vi "StaticCalibration2.vi"(0 "SENSOR":T1, 11 "error in (no error)":errorcluster caption="错误输入（无错误）") -> (4 "Vres":dbl, 6 "Angle out":dbl, 8 "Vres_FD":i32, 10 "OK？":bool, 15 "error out":errorcluster caption="错误输出")   [LabVIEW 2020]
doc: "该模板用于创建子VI。"
uses:
  Global_Variable/Global.vi
  <userlib>/DAQNavi Polymorphic VI/create/DAQNavi Create Channel.vi
  <userlib>/DAQNavi Polymorphic VI/create/DAQNavi Create Channel(CI-PulseWidth).vi
  <userlib>/DAQNavi Polymorphic VI/read/DAQNavi Read.vi
  <userlib>/DAQNavi Polymorphic VI/read/DAQNavi Read (Counter Pulse Width 1Chan 1Samp).vi
  <userlib>/DAQNavi Polymorphic VI/configure/task/DAQNavi Clear Task.vi
  <userlib>/_MGI/1D Array/MGI Average.vi
  <userlib>/_MGI/1D Array/MGI Average/MGI Average (DBL[]).vi
panel:
  out "T2(%)":dbl
  out "T1(%)":dbl
  out "S(%)":dbl
  out "P(%)":dbl
  out "T2ROC_1+T2ROC_2":i32
  out "T1ROC_1+T1ROC_2":i32
  out "PROC_1":i32
  out "T2ROC_1":i32
  out "T1ROC_1":i32
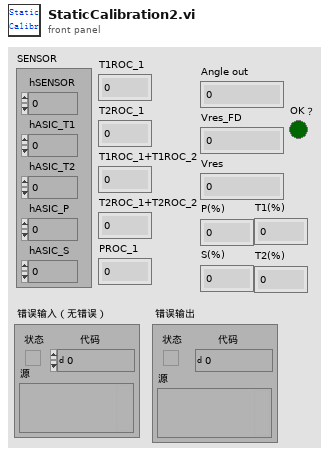
[diagram p1: front panel]
types:
  T1 = cluster{"hSENSOR":i32, "hASIC_T1":i32, "hASIC_T2":i32, "hASIC_P":i32, "hASIC_S":i32}
  T2 = cluster{"主信号":cluster{"单位":string, "下限":dbl, "上限":dbl}, "副信号":cluster{"单位":string, "下限":dbl, "上限":dbl}, "主副和":cluster{"单位":string, "下限":dbl, "上限":dbl}, "主副差":cluster{"单位":string, "下限":dbl, "上限":dbl}, "Vres":cluster{"单位":string, "下限":dbl, "上限":dbl}}
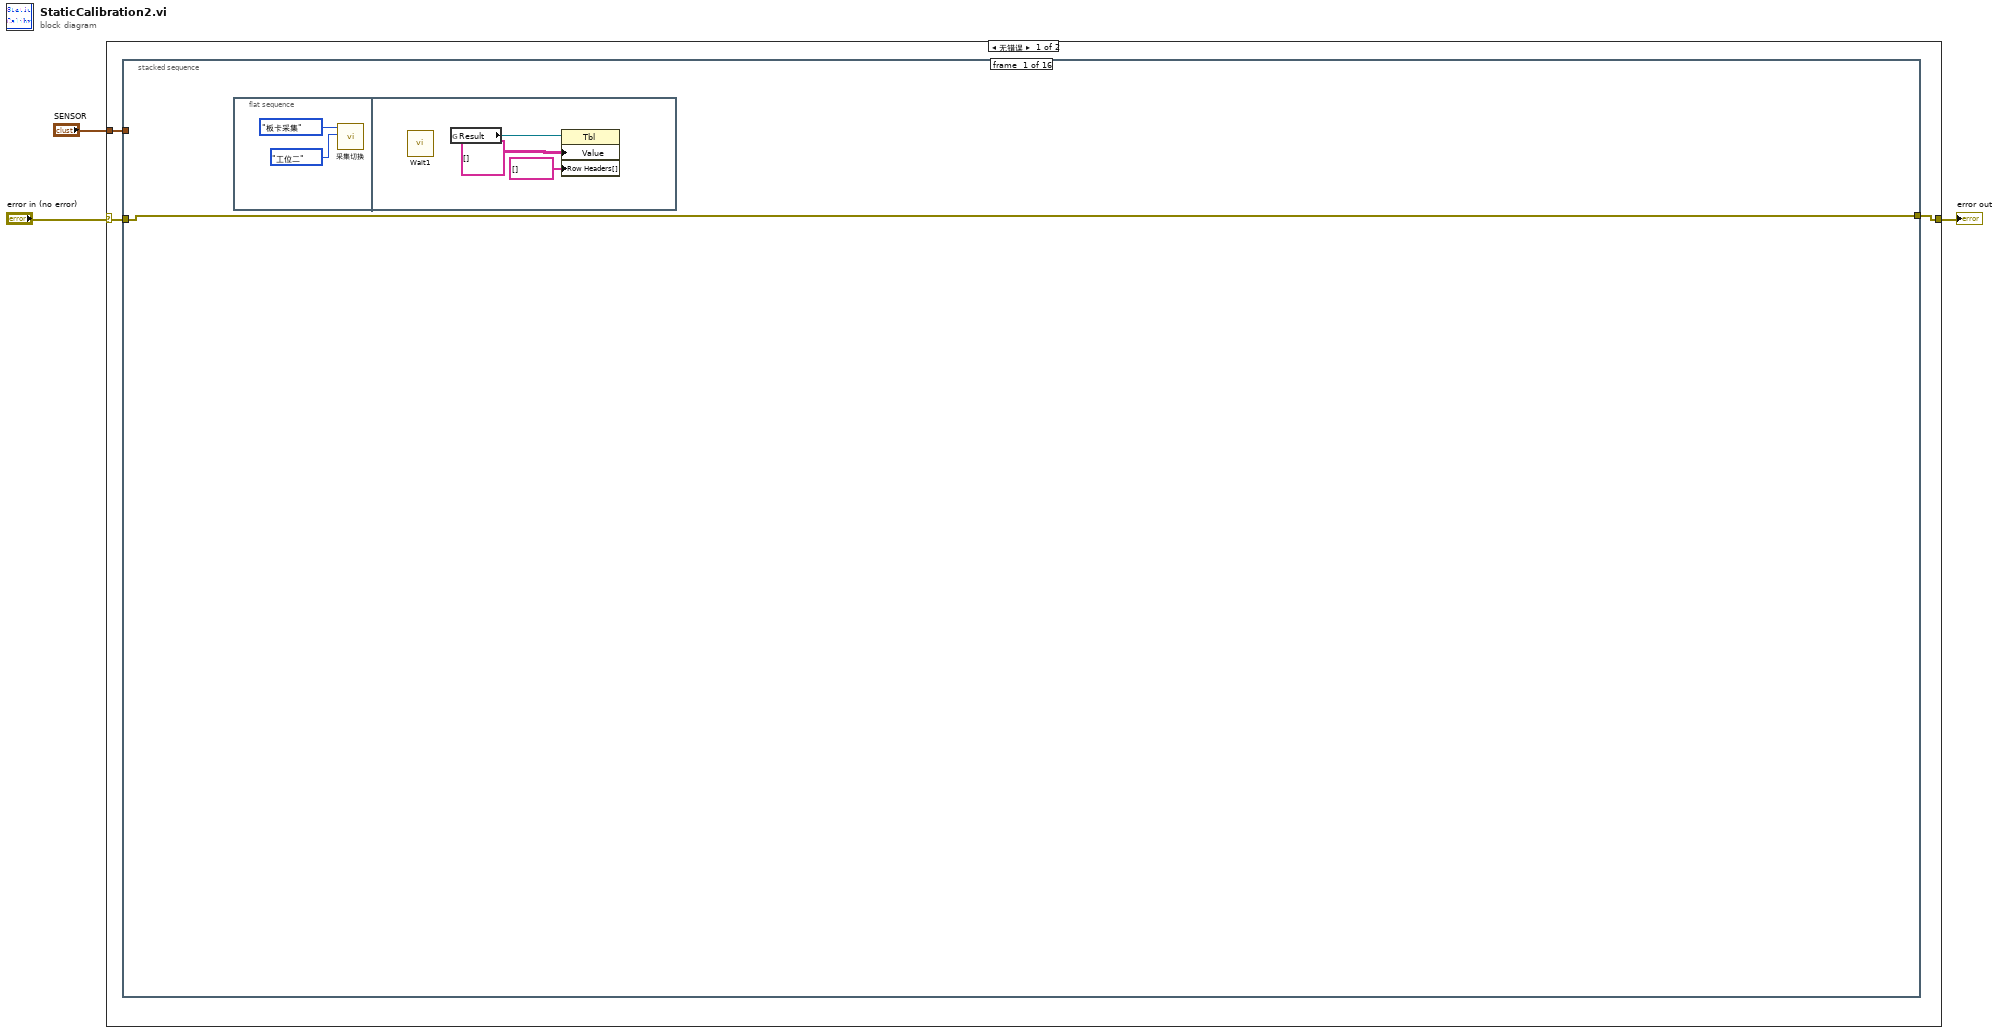
[diagram p0: block diagram]
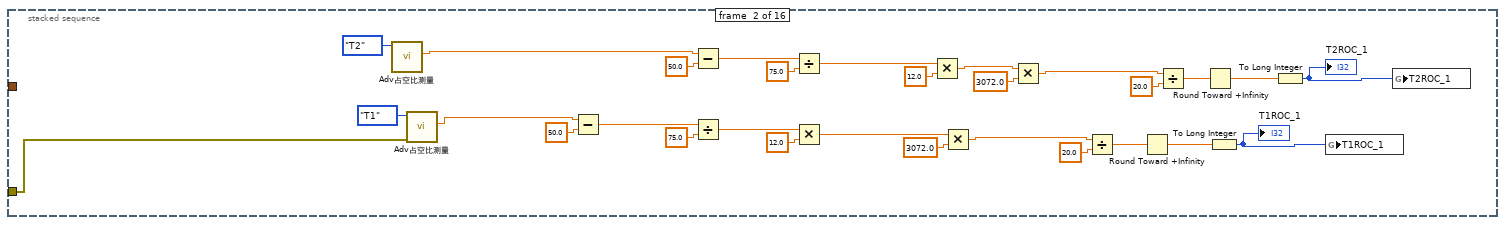
[diagram p2: hidden frame]
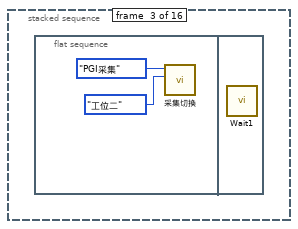
[diagram p3: hidden frame]
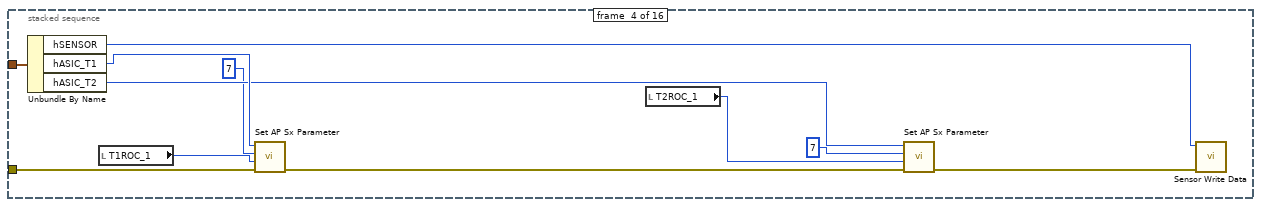
[diagram p4: hidden frame]
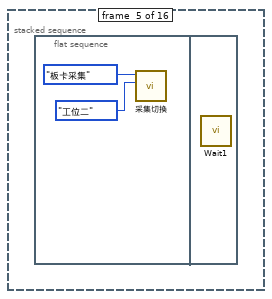
[diagram p5: hidden frame]
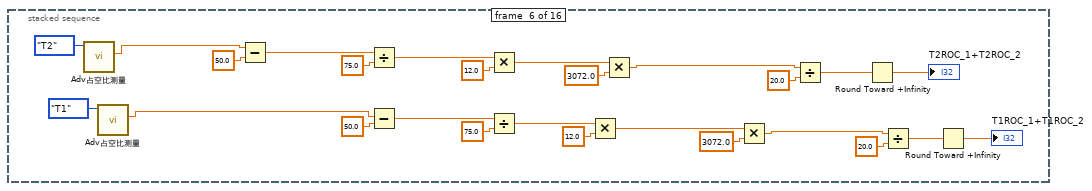
[diagram p6: hidden frame]
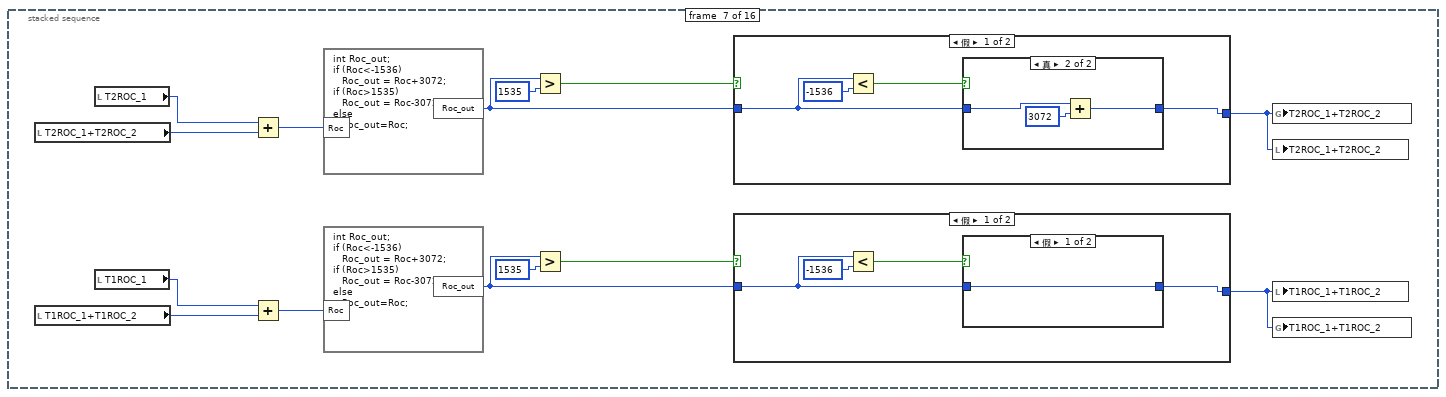
[diagram p7: hidden frame]
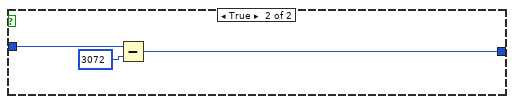
[diagram p9: hidden frame]
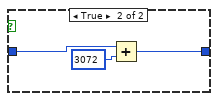
[diagram p10: hidden frame]
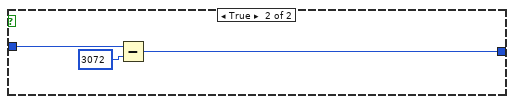
[diagram p11: hidden frame]
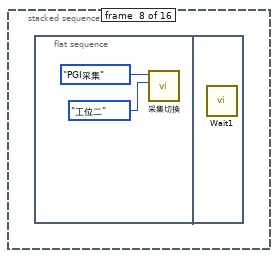
[diagram p12: hidden frame]
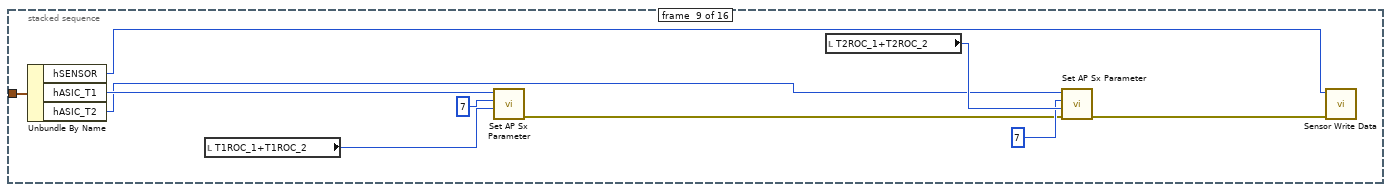
[diagram p13: hidden frame]
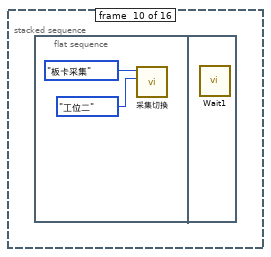
[diagram p14: hidden frame]
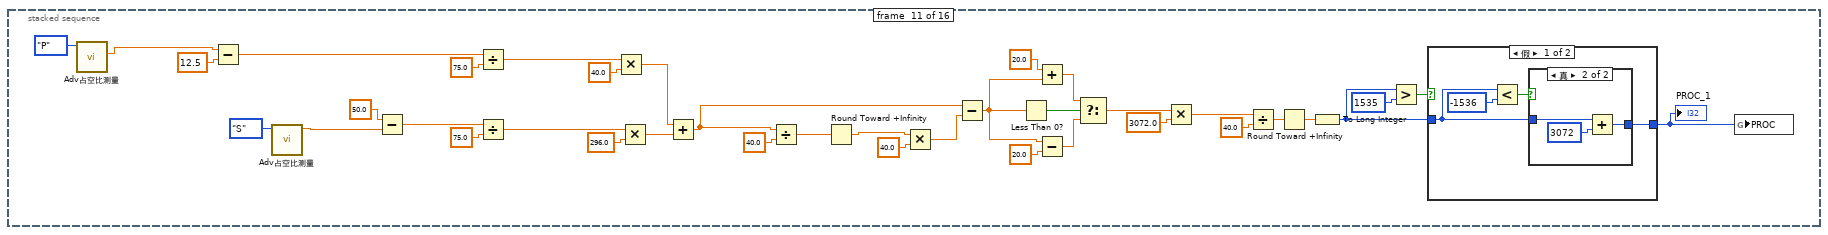
[diagram p15: hidden frame]
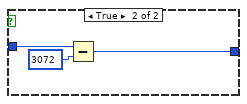
[diagram p17: hidden frame]
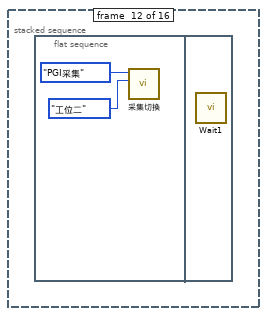
[diagram p18: hidden frame]
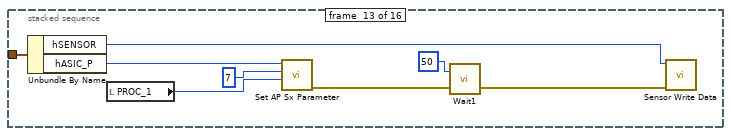
[diagram p19: hidden frame]
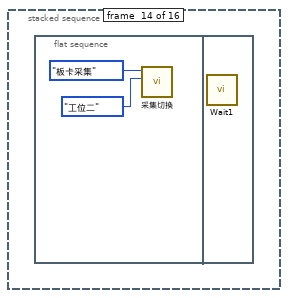
[diagram p20: hidden frame]
diagram:
  n1 = case shown="无错误" "error in (no error)" {
    selector: "error in (no error)" -> [w5 w304]
    tunnel: [w4 w304] -> w2
    tunnel: "SENSOR" -> [w6 _]
    frame No Error {
      n2 = stacked-sequence {
        tunnel: w6 -> [_ _ _ w52 _ _ _ _ w129 _ _ _ w186 _ _ _]
        tunnel: w5 -> [w7 w13 _ w44 _ _ _ _ _ _ _ _ _ _ _ _]
        tunnel: [w7 _ _ _ _ _ _ _ _ _ _ _ _ _ _ _] -> w4
        frame #0 {
          n3 = flat-sequence {
            frame #0 {
              n4 = call "采集切换.vi"("工位"=enum16{"工位一", "工位二"}."工位二", "采集方式"=enum16{"板卡采集", "PGI采集"}."板卡采集") -> ()  [unwired: 10 in]
            }
            frame #1 {
              n5 = call "Wait1.vi"() -> ()  [unwired: 3 in, 1 out]
              n6 = global read "Global.vi" "Result"() -> (w12:refnum<vi>)
              n7 = property class="Tbl"(reference=w12, "Value"=string[][] [] ("值"), "Row Headers[]"=string[] [] ("行首字符串[]")) -> ()  [unwired: 1 in, 2 out]
            }
          }
        }
        frame #1 {
          n8 = call "Adv占空比测量.vi"("通道"=enum16{"T1", "T2", "P", "S"}."T2") -> ("占空比2"=w16:dbl)  [unwired: 5 in, 4 out]
          n9 = call "Adv占空比测量.vi"("通道"=enum16{"T1", "T2", "P", "S"}."T1", "error in (no error)"=w13) -> ("占空比2"=w14:dbl)  [unwired: 4 in, 4 out]
          n10 = Subtract(x=w14, y=50.0) -> (x-y=w40:dbl)
          n11 = Subtract(x=w16, y=50.0) -> (x-y=w25:dbl)
          n12 = Divide(x=w40, y=75.0) -> (x/y=w38:dbl)
          n13 = Divide(x=w25, y=75.0) -> (x/y=w27:dbl)
          n14 = Multiply(x=w38, y=12.0) -> (x*y=w36:dbl)
          n15 = Multiply(x=w27, y=12.0) -> (x*y=w29:dbl)
          n16 = Multiply(x=w36, y=3072.0) -> (x*y=w34:dbl)
          n17 = Multiply(x=w29, y=3072.0) -> (x*y=w31:dbl)
          n18 = Divide(x=w34, y=20.0) -> (x/y=w23:dbl)
          n19 = Round Toward +Infinity(x=w23) -> (ceil(x): smallest int >= x=w21:dbl)
          n20 = Divide(x=w31, y=20.0) -> (x/y=w22:dbl)
          n21 = Round Toward +Infinity(x=w22) -> (ceil(x): smallest int >= x=w20:dbl)
          n22 = To Long Integer(number=w21) -> (32bit integer=w18:i32)
          "T1ROC_1" <- w18
          n23 = To Long Integer(number=w20) -> (32bit integer=w19:i32)
          "T2ROC_1" <- w19
          n24 = global write "Global.vi" "T1ROC_1"(w18) -> ()
          n25 = global write "Global.vi" "T2ROC_1"(w19) -> ()
        }
        frame #2 {
          n26 = flat-sequence {
            frame #0 {
              n27 = call "采集切换.vi"("工位"=enum16{"工位一", "工位二"}."工位二", "采集方式"=enum16{"板卡采集", "PGI采集"}."PGI采集") -> ()  [unwired: 10 in]
            }
            frame #1 {
              n28 = call "Wait1.vi"() -> ()  [unwired: 3 in, 1 out]
            }
          }
        }
        frame #3 {
          n29 = Unbundle By Name(w52) -> ("hSENSOR"=w49:i32, "hASIC_T1"=w51:i32, "hASIC_T2"=w50:i32)
          n30 = local read "T1ROC_1"() -> (w53:i32)
          n31 = call "Set AP Sx Parameter.vi"("error in (no error)"=w44, "para2"=w53, "asicBitsName"=7, "asicHandle"=w51) -> ("error out"=w46:errorcluster)  [unwired: 6 in, 1 out]
          n32 = local read "T2ROC_1"() -> (w54:i32)
          n33 = call "Set AP Sx Parameter.vi"("error in (no error)"=w46, "para2"=w54, "asicBitsName"=7, "asicHandle"=w50) -> ("error out"=w45:errorcluster)  [unwired: 6 in, 1 out]
          n34 = call "Sensor Write Data.vi"("error in (no error)"=w45, "sensorHandle"=w49) -> ()  [unwired: 8 in, 2 out]
        }
        frame #4 {
          n35 = flat-sequence {
            frame #0 {
              n36 = call "采集切换.vi"("工位"=enum16{"工位一", "工位二"}."工位二", "采集方式"=enum16{"板卡采集", "PGI采集"}."板卡采集") -> ()  [unwired: 10 in]
            }
            frame #1 {
              n37 = call "Wait1.vi"() -> ()  [unwired: 3 in, 1 out]
            }
          }
        }
        frame #5 {
          n38 = call "Adv占空比测量.vi"("通道"=enum16{"T1", "T2", "P", "S"}."T2") -> ("占空比2"=w60:dbl)  [unwired: 5 in, 4 out]
          n39 = call "Adv占空比测量.vi"("通道"=enum16{"T1", "T2", "P", "S"}."T1") -> ("占空比2"=w59:dbl)  [unwired: 5 in, 4 out]
          n40 = Subtract(x=w60, y=50.0) -> (x-y=w82:dbl)
          n41 = Divide(x=w82, y=75.0) -> (x/y=w81:dbl)
          n42 = Subtract(x=w59, y=50.0) -> (x-y=w75:dbl)
          n43 = Multiply(x=w81, y=12.0) -> (x*y=w80:dbl)
          n44 = Divide(x=w75, y=75.0) -> (x/y=w76:dbl)
          n45 = Multiply(x=w76, y=12.0) -> (x*y=w77:dbl)
          n46 = Multiply(x=w80, y=3072.0) -> (x*y=w79:dbl)
          n47 = Multiply(x=w77, y=3072.0) -> (x*y=w78:dbl)
          n48 = Divide(x=w79, y=20.0) -> (x/y=w73:dbl)
          n49 = Round Toward +Infinity(x=w73) -> (ceil(x): smallest int >= x=→"T2ROC_1+T2ROC_2":dbl)
          n50 = Divide(x=w78, y=20.0) -> (x/y=w74:dbl)
          n51 = Round Toward +Infinity(x=w74) -> (ceil(x): smallest int >= x=→"T1ROC_1+T1ROC_2":dbl)
        }
        frame #6 {
          n52 = local read "T2ROC_1+T2ROC_2"() -> (w85:i32)
          n53 = local read "T1ROC_1+T1ROC_2"() -> (w86:i32)
          n54 = local read "T2ROC_1"() -> (w93:i32)
          n55 = local read "T1ROC_1"() -> (w94:i32)
          n56 = Add(x=w93, y=w85) -> (x+y=w95:i32)
          n57 = Add(x=w94, y=w86) -> (x+y=w96:i32)
          n58 = formula code="int Roc_out;\nif (Roc<-1536)\n   Roc_out = Roc+3072;\nif (Roc>1535)\n   Roc_out = Roc-3072;\nelse\n   Roc_out=Roc;"("Roc"=w95) -> ("Roc_out"=w87:i32)
          n59 = formula code="int Roc_out;\nif (Roc<-1536)\n   Roc_out = Roc+3072;\nif (Roc>1535)\n   Roc_out = Roc-3072;\nelse\n   Roc_out=Roc;"("Roc"=w96) -> ("Roc_out"=w90:i32)
          n60 = Greater?(x=w87, y=1535) -> (0:w88:bool)
          n61 = Greater?(x=w90, y=1535) -> (0:w91:bool)
          n62 = case shown="假" w88 {
            tunnel: w87 -> [w98 w106]
            tunnel: [w97 w105] -> w83
            frame False {
              n63 = Less?(x=w98, y=-1536) -> (x < y?=w99:bool)
              n64 = case shown="真" w99 {
                tunnel: w98 -> [w101 w104]
                tunnel: [w101 w102] -> w97
                frame False {
                }
                frame True {
                  n65 = Add(x=w104, y=3072) -> (x+y=w102:i32)
                }
              }
            }
            frame True {
              n66 = Subtract(x=w106, y=3072) -> (x-y=w105:i32)
            }
          }
          n67 = case shown="假" w91 {
            tunnel: w90 -> [w109 w117]
            tunnel: [w108 w116] -> w84
            frame False {
              n68 = Less?(x=w109, y=-1536) -> (x < y?=w110:bool)
              n69 = case shown="假" w110 {
                tunnel: w109 -> [w112 w115]
                tunnel: [w112 w113] -> w108
                frame False {
                }
                frame True {
                  n70 = Add(x=w115, y=3072) -> (x+y=w113:i32)
                }
              }
            }
            frame True {
              n71 = Subtract(x=w117, y=3072) -> (x-y=w116:i32)
            }
          }
          n72 = global write "Global.vi" "T2ROC_1+T2ROC_2"(w83) -> ()
          n73 = local write "T2ROC_1+T2ROC_2"(w83) -> ()
          n74 = local write "T1ROC_1+T1ROC_2"(w84) -> ()
          n75 = global write "Global.vi" "T1ROC_1+T1ROC_2"(w84) -> ()
        }
        frame #7 {
          n76 = flat-sequence {
            frame #0 {
              n77 = call "采集切换.vi"("工位"=enum16{"工位一", "工位二"}."工位二", "采集方式"=enum16{"板卡采集", "PGI采集"}."PGI采集") -> ()  [unwired: 10 in]
            }
            frame #1 {
              n78 = call "Wait1.vi"() -> ()  [unwired: 3 in, 1 out]
            }
          }
        }
        frame #8 {
          n79 = Unbundle By Name(w129) -> ("hSENSOR"=w126:i32, "hASIC_T1"=w128:i32, "hASIC_T2"=w127:i32)
          n80 = local read "T1ROC_1+T1ROC_2"() -> (w125:i32)
          n81 = call "Set AP Sx Parameter.vi"("para2"=w125, "asicBitsName"=7, "asicHandle"=w128) -> ("error out"=w122:errorcluster)  [unwired: 7 in, 1 out]
          n82 = local read "T2ROC_1+T2ROC_2"() -> (w130:i32)
          n83 = call "Set AP Sx Parameter.vi"("error in (no error)"=w122, "para2"=w130, "asicBitsName"=7, "asicHandle"=w127) -> ("error out"=w121:errorcluster)  [unwired: 6 in, 1 out]
          n84 = call "Sensor Write Data.vi"("error in (no error)"=w121, "sensorHandle"=w126) -> ()  [unwired: 8 in, 2 out]
        }
        frame #9 {
          n85 = flat-sequence {
            frame #0 {
              n86 = call "采集切换.vi"("工位"=enum16{"工位一", "工位二"}."工位二", "采集方式"=enum16{"板卡采集", "PGI采集"}."板卡采集") -> ()  [unwired: 10 in]
            }
            frame #1 {
              n87 = call "Wait1.vi"() -> ()  [unwired: 3 in, 1 out]
            }
          }
        }
        frame #10 {
          n88 = call "Adv占空比测量.vi"("通道"=enum16{"T1", "T2", "P", "S"}."P") -> ("占空比2"=w136:dbl)  [unwired: 5 in, 4 out]
          n89 = Subtract(x=w136, y=12.5) -> (x-y=w169:dbl)
          n90 = call "Adv占空比测量.vi"("通道"=enum16{"T1", "T2", "P", "S"}."S") -> ("占空比1"=w134:dbl)  [unwired: 5 in, 4 out]
          n91 = Subtract(x=50.0, y=w134) -> (x-y=w163:dbl)
          n92 = Divide(x=w169, y=75.0) -> (x/y=w167:dbl)
          n93 = Divide(x=w163, y=75.0) -> (x/y=w161:dbl)
          n94 = Multiply(x=w167, y=40.0) -> (x*y=w165:dbl)
          n95 = Multiply(x=w161, y=296.0) -> (x*y=w159:dbl)
          n96 = Add(x=w165, y=w159) -> (x+y=w153:dbl)
          n97 = Divide(x=w153, y=40.0) -> (x/y=w157:dbl)
          n98 = Round Toward +Infinity(x=w157) -> (ceil(x): smallest int >= x=w155:dbl)
          n99 = Multiply(x=w155, y=40.0) -> (x*y=w154:dbl)
          n100 = Subtract(x=w153, y=w154) -> (x-y=w149:dbl)
          n101 = Less Than 0?(x=w149) -> (x < 0?=w148:bool)
          n102 = Add(x=20.0, y=w149) -> (x+y=w151:dbl)
          n103 = Subtract(x=w149, y=20.0 ("x")) -> (x-y=w147:dbl)
          n104 = Select(t=w151, s=w148, f=w147) -> (s? t:f=w146:dbl)
          n105 = Multiply(x=w146, y=3072.0) -> (x*y=w144:dbl)
          n106 = Divide(x=w144, y=40.0) -> (x/y=w139:dbl)
          n107 = Round Toward +Infinity(x=w139) -> (ceil(x): smallest int >= x=w138:dbl)
          n108 = To Long Integer(number=w138) -> (32bit integer=w142:i32)
          n109 = Greater?(x=w142, y=1535) -> (0:w140:bool)
          n110 = case shown="假" w140 {
            tunnel: w142 -> [w172 w180]
            tunnel: [w171 w179] -> w137
            frame False {
              n111 = Less?(x=w172, y=-1536) -> (x < y?=w173:bool)
              n112 = case shown="真" w173 {
                tunnel: w172 -> [w175 w178]
                tunnel: [w175 w176] -> w171
                frame False {
                }
                frame True {
                  n113 = Add(x=w178, y=3072) -> (x+y=w176:i32)
                }
              }
            }
            frame True {
              n114 = Subtract(x=w180, y=3072) -> (x-y=w179:i32)
            }
          }
          "PROC_1" <- w137
          n115 = global write "Global.vi" "PROC"(w137) -> ()
        }
        frame #11 {
          n116 = flat-sequence {
            frame #0 {
              n117 = call "采集切换.vi"("工位"=enum16{"工位一", "工位二"}."工位二", "采集方式"=enum16{"板卡采集", "PGI采集"}."PGI采集") -> ()  [unwired: 10 in]
            }
            frame #1 {
              n118 = call "Wait1.vi"() -> ()  [unwired: 3 in, 1 out]
            }
          }
        }
        frame #12 {
          n119 = Unbundle By Name(w186) -> ("hSENSOR"=w185:i32, "hASIC_P"=w184:i32)
          n120 = local read "PROC_1"() -> (w189:i32)
          n121 = call "Set AP Sx Parameter.vi"("para2"=w189, "asicBitsName"=7, "asicHandle"=w184) -> ("error out"=w191:errorcluster)  [unwired: 7 in, 1 out]
          n122 = call "Wait1.vi"("error in (no error)"=w191, "Wait（150ms）"=u32 50) -> ("error out"=w190:errorcluster)  [unwired: 1 in]
          n123 = call "Sensor Write Data.vi"("error in (no error)"=w190, "sensorHandle"=w185) -> ()  [unwired: 8 in, 2 out]
        }
        frame #13 {
          n124 = flat-sequence {
            frame #0 {
              n125 = call "采集切换.vi"("工位"=enum16{"工位一", "工位二"}."工位二", "采集方式"=enum16{"板卡采集", "PGI采集"}."板卡采集") -> ()  [unwired: 10 in]
            }
            frame #1 {
              n126 = call "Wait1.vi"() -> ()  [unwired: 3 in, 1 out]
            }
          }
        }
        frame #14 {
          n127 = call "Adv占空比测量.vi"("通道"=enum16{"T1", "T2", "P", "S"}."S") -> (4:"占空比1"=w194:dbl[], 7:"占空比1"=w210:dbl)  [unwired: 5 in, 3 out]
          "S(%)" <- w210
          n128 = call "Adv占空比测量.vi"("通道"=enum16{"T1", "T2", "P", "S"}."P") -> (5:"占空比2"=w195:dbl[], 8:"占空比2"=w212:dbl)  [unwired: 5 in, 3 out]
          "P(%)" <- w212
          n129 = call "Adv占空比测量.vi"("通道"=enum16{"T1", "T2", "P", "S"}."T2") -> (5:"占空比2"=w197:dbl[], 8:"占空比2"=→"T2(%)":dbl)  [unwired: 5 in, 3 out]
          n130 = call "Adv占空比测量.vi"("通道"=enum16{"T1", "T2", "P", "S"}."T1") -> (5:"占空比2"=w196:dbl[], 8:"占空比2"=→"T1(%)":dbl)  [unwired: 5 in, 3 out]
          n131 = call <vilib>:"Application Directory.vi"() -> ("Application Directory"=w206:path)
          n132 = call "Calc_Vres.vi"("S_Data in"=w210, "P_Data in"=w212) -> ("Vres_FD"=→"Vres_FD":i32, "Vres"=→"Vres":dbl, "Angle out"=→"Angle out":dbl)  [unwired: 7 in]
          n133 = call <vilib>:"Application Directory.vi"() -> ("Application Directory"=w207:path)
          n134 = Build Path(base path=w206, name or relative path="P.txt") -> (appended path=w205:path)
          n135 = Build Path(base path=w207, name or relative path="T2.txt") -> (appended path=w208:path)
          n136 = call "导出曲线数组.vi"("file path (dialog if empty)"=w205, "数组"=w195) -> ()  [unwired: 10 in]
          n137 = call "导出曲线数组.vi"("file path (dialog if empty)"=w208, "数组"=w197) -> ()  [unwired: 10 in]
          n138 = call <vilib>:"Application Directory.vi"() -> ("Application Directory"=w201:path)
          n139 = call <vilib>:"Application Directory.vi"() -> ("Application Directory"=w200:path)
          n140 = Build Path(base path=w201, name or relative path="S.txt") -> (appended path=w202:path)
          n141 = Build Path(base path=w200, name or relative path="T1.txt") -> (appended path=w199:path)
          n142 = call "导出曲线数组.vi"("file path (dialog if empty)"=w202, "数组"=w194) -> ()  [unwired: 10 in]
          n143 = call "导出曲线数组.vi"("file path (dialog if empty)"=w199, "数组"=w196) -> ()  [unwired: 10 in]
        }
        frame #15 {
          (unwired) "96.000"
          n144 = local read "T1(%)"() -> (w256:dbl)
          n145 = local read "T2(%)"() -> (w255:dbl)
          n146 = global read "Global.vi" "静态标定判定"() -> (w253:T2)
          n147 = Add(x=w256, y=w255) -> (x+y=w294:dbl)
          n148 = Subtract(x=w256, y=w255) -> (x-y=w259:dbl)
          n149 = Unbundle By Name(w253) -> ("主信号.上限"=w238:dbl, "主信号.下限"=w240:dbl)
          n150 = Unbundle By Name(w253) -> ("主副和.上限"=w231:dbl, "主副和.下限"=w232:dbl)
          n151 = Unbundle By Name(w253) -> ("主副差.上限"=w229:dbl, "主副差.下限"=w230:dbl)
          n152 = Unbundle By Name(w253) -> ("副信号.上限"=w235:dbl, "副信号.下限"=w236:dbl)
          n153 = Unbundle By Name(w253) -> ("Vres.上限"=w227:dbl, "Vres.下限"=w228:dbl)
          n154 = local read "Vres"() -> (w298:dbl)
          n155 = Absolute Value(x=w259) -> (abs(x)=w254:dbl)
          n156 = In Range and Coerce(upper limit=w227, x=w298, lower limit=w228) -> (In Range?=w251:bool)  [unwired: 1 out]
          n157 = In Range and Coerce(upper limit=w238, x=w256, lower limit=w240) -> (In Range?=w270:bool)  [unwired: 1 out]
          n158 = In Range and Coerce(upper limit=w231, x=w294, lower limit=w232) -> (In Range?=w268:bool)  [unwired: 1 out]
          n159 = In Range and Coerce(upper limit=w229, x=w254, lower limit=w230) -> (In Range?=w252:bool)  [unwired: 1 out]
          n160 = In Range and Coerce(upper limit=w235, x=w255, lower limit=w236) -> (In Range?=w269:bool)  [unwired: 1 out]
          n161 = Build Array(w270, w269, w268, w252, w251) -> (w267:bool[])
          n162 = Select(t="OK", s=w251, f="NG") -> (s? t:f=w280:string)
          n163 = Select(t="OK", s=w270, f="NG") -> (s? t:f=w291:string)
          n164 = Select(t="OK", s=w268, f="NG") -> (s? t:f=w282:string)
          n165 = Select(t="OK", s=w252, f="NG") -> (s? t:f=w263:string)
          n166 = Select(t="OK", s=w269, f="NG") -> (s? t:f=w290:string)
          n167 = And Array Elements(Boolean array=w267) -> (logical AND=→"OK？":bool)
          n168 = Number To Fractional String(number=w298, precision (6)=i16 3 ("精度(6)")) -> (F-format string=w277:string)  [unwired: 2 in]
          n169 = Number To Fractional String(number=w227, precision (6)=i16 3 ("精度(6)")) -> (F-format string=w221:string)  [unwired: 2 in]
          n170 = Number To Fractional String(number=w228, precision (6)=i16 3 ("精度(6)")) -> (F-format string=w222:string)  [unwired: 2 in]
          n171 = Number To Fractional String(number=w238, precision (6)=i16 3 ("精度(6)")) -> (F-format string=w237:string)  [unwired: 2 in]
          n172 = Number To Fractional String(number=w240, precision (6)=i16 3 ("精度(6)")) -> (F-format string=w239:string)  [unwired: 2 in]
          n173 = Number To Fractional String(number=w231, precision (6)=i16 3 ("精度(6)")) -> (F-format string=w225:string)  [unwired: 2 in]
          n174 = Number To Fractional String(number=w232, precision (6)=i16 3 ("精度(6)")) -> (F-format string=w226:string)  [unwired: 2 in]
          n175 = Number To Fractional String(number=w229, precision (6)=i16 3 ("精度(6)")) -> (F-format string=w223:string)  [unwired: 2 in]
          n176 = Number To Fractional String(number=w230, precision (6)=i16 3 ("精度(6)")) -> (F-format string=w224:string)  [unwired: 2 in]
          n177 = Number To Fractional String(number=w235, precision (6)=i16 3 ("精度(6)")) -> (F-format string=w233:string)  [unwired: 2 in]
          n178 = Number To Fractional String(number=w236, precision (6)=i16 3 ("精度(6)")) -> (F-format string=w234:string)  [unwired: 2 in]
          n179 = Number To Fractional String(number=w256, precision (6)=i16 3 ("精度(6)")) -> (F-format string=w293:string)  [unwired: 2 in]
          n180 = Number To Fractional String(number=w294, precision (6)=i16 3 ("精度(6)")) -> (F-format string=w281:string)  [unwired: 2 in]
          n181 = Number To Fractional String(number=w254, precision (6)=i16 3 ("精度(6)")) -> (F-format string=w264:string)  [unwired: 2 in]
          n182 = Number To Fractional String(number=w255, precision (6)=i16 3 ("精度(6)")) -> (F-format string=w287:string)  [unwired: 2 in]
          n183 = Build Array(w222, w277, w221, "%", w280) -> (w272:string[])
          n184 = Build Array(w239, w293, w237, "%", w291) -> (w275:string[])
          n185 = Build Array(w234, w287, w233, "%", w290) -> (w274:string[])
          n186 = Build Array(w226, w281, w225, "%", w282) -> (w273:string[])
          n187 = Build Array(w224, w264, w223, "%", w263) -> (w257:string[])
          n188 = global read "Global.vi" "Result"() -> (w303:refnum<vi>)
          n189 = Build Array(string[] [""] ("元素"), w275, w274, w273, w257, w272) -> (w271:string[][])
          n190 = property class="Tbl"(reference=w303, "Row Headers[]"=string[] ["静态标定", "T1", "T2", "T1+T2", "T1-T2", "Vres"] ("行首字符串[]"), "Value"=w271) -> ()  [unwired: 1 in, 2 out]
        }
      }
    }
    frame Error {
    }
  }
  "error out" <- w2
